vi "grabImages.vi"(8 "error in (no error)":errorcluster, 10 "how many images":i32=50, 11 "WebSocket in":refnum<class "WebSocket.lvclass">) -> (0 "error out":errorcluster)   [LabVIEW 2018]
doc: "The Acquire Most Recent Image example acquires images continuously and displays the images in an image control using a grab acquisition. It uses the <B>Last New</B> acquisition mode to get the most recent image to avoid waiting for a new image to be acquired."
uses:
  <vilib>/MediaMongrels Ltd/WebSockets/WebSockets/WebSocket/WebSocket.lvclass
  <vilib>/vision/driver/IMAQdx.llb/IMAQdx Buffer Number Mode.ctl
  <vilib>/vision/driver/NI_Vision_Acquisition_Software.lvlib
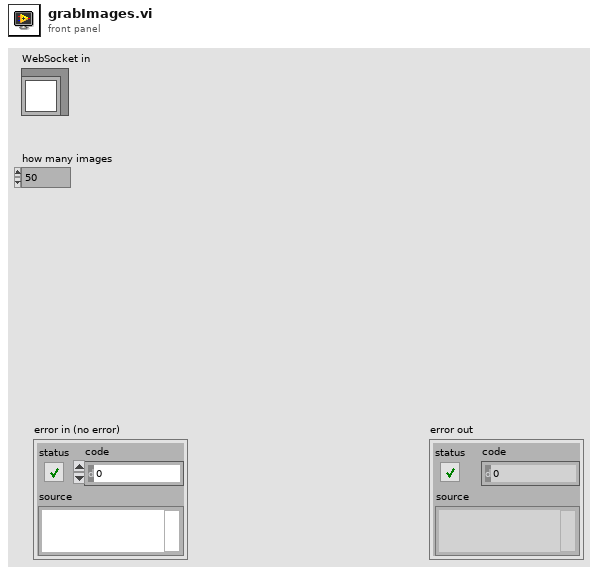
[diagram p1: front panel]
types:
  T1 = typedef "IMAQdx.ctl" = refnum<k21>
  T2 = typedef "IMAQ Image.ctl" = refnum<image>
  T3 = typedef "NI_Vision_Acquisition_Software.lvlib/IMAQdx Buffer Number Mode.ctl" = enum32{"Next", "Last", "Buffer Number", "Every", "Last New"}
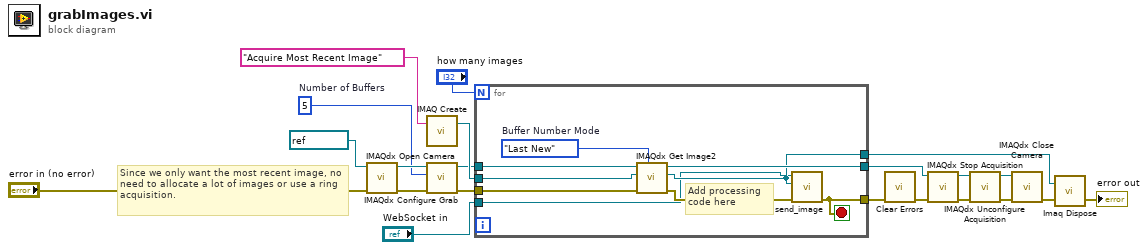
[diagram p0: block diagram]
diagram:
  w9 = u32 5  # Number of Buffers
  # "Since we only want the most recent image, no need to allocate a lot of images or use a ring acquisition."
  n1 = call <vilib>:"IMAQdx Open Camera.vi"("error in"="error in (no error)", "Session In"=refnum<k21> "cam0" ("Camera Name")) -> ("error out"=w8:errorcluster, "Session Out"=w10:T1)  [unwired: 1 in, 7 out]
  n2 = call "IMAQ Create"("Image Name"="Acquire Most Recent Image") -> ("New Image"=w21:T2)  [unwired: 3 in, 2 out]
  n3 = call <vilib>:"IMAQdx Configure Grab.vi"("error in"=w8, "Number of Buffers"=w9, "Session In"=w10) -> ("error out"=w6:errorcluster, "Session Out"=w7:T1)  [unwired: 7 in]
  n4 = for {
    N: "how many images" -> [_]
    tunnel: [w26] -> w18
    tunnel: w6 -> [w29]
    tunnel: w7 -> [w30]
    tunnel: [w22] -> w19
    tunnel: w21 -> [w28]
    tunnel: [w24] -> w11
    tunnel: "WebSocket in" -> [w23]
    stop <- w22 stop-if-true
    w27 = IMAQdx_Buffer_Number_Mode."Last New"  # Buffer Number Mode
    # "Add processing code here"
    n5 = call <vilib>:"IMAQdx Get Image2.vi"("Buffer Number Mode (Next)"=w27, "error in"=w29, "Image In"=w28, "Session In"=w30) -> ("error out"=w25:errorcluster, "Image Out"=w24:T2, "Session Out"=w26:T1)  [unwired: 4 in, 1 out]
    n6 = call "send_image.vi"("error in (no error)"=w25, "img in"=w24, "WebSocket in"=w23) -> ("error out"=w22:errorcluster)  [unwired: 7 in, 1 out]
  }
  n7 = call <vilib>:"Clear Errors.vi"("error in (no error)"=w19) -> ("error out"=w3:errorcluster)  [unwired: 5 in, 1 out]
  n8 = call <vilib>:"IMAQdx Stop Acquisition.vi"("error in"=w3, "Session In"=w18) -> ("error out"=w14:errorcluster, "Session Out"=w15:T1)  [unwired: 8 out]
  n9 = call <vilib>:"IMAQdx Unconfigure Acquisition.vi"("error in"=w14, "Session In"=w15) -> ("error out"=w17:errorcluster, "Session Out"=w16:T1)  [unwired: 8 out]
  n10 = call <vilib>:"IMAQdx Close Camera.vi"("error in"=w17, "Session In"=w16) -> ("error out"=w13:errorcluster)  [unwired: 9 out]
  n11 = call "Imaq Dispose"("Image"=w11, "error in (no error)"=w13) -> ("error out"=→"error out":errorcluster)  [unwired: 4 in]
